vi "RF Rec Generate Waveform.vi"   [LabVIEW 2018]
doc: "Creates a waveform to send to a device for generation."
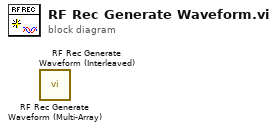
[diagram p0: block diagram]
diagram:
  n1 = call "RF Rec Generate Waveform (Multi-Array).vi"() -> ()  [unwired: 12 in, 4 out]
  n2 = call "RF Rec Generate Waveform (Interleaved).vi"() -> ()  [unwired: 13 in, 3 out]
